vi "Sequencer.RF.vi"() -> ()   [LabVIEW 2014]
uses:
  <vilib>/Analysis/NI_AALPro.lvlib
panel:
  in  "Trigger":bool
  in  "Parameter":u16(ring) items=["Frequency (MHz)", "Amplitude (dBm)", "Phase (Pi)"]
  in  "Oscillators":u32(ring) items=["Agilent 1", "Agilent 2"]
  out "Counts":u32[](array[numeric])
  in  "Threshold":dbl=9.0
  out "CompiledSequence":string="#DopplerCooling\r\n0.9 10100000 00000000 00000000\r\n\r\n#Pump\r\n0.3 01000000 00000000 00000000\r\n\r\n#Pulsed\r\n0.2 00100000 00000000 00000000\r\n0.4 00000100 00000000 00000000\r\n0.2 00000000 10000000 00000000\r\n0.2 01000000 00000000 01000000\n"
  out "ChapterNames":string[](array[string])
  out "ChapterPositions":u32[](array[numeric])
  in  "Scan":enum32{"Time", "RF"}(tab)=enum."RF"
  out "Now (us)":dbl=1.0 format="%.2f"
  in  "Step (us)":dbl=1.0 format="%.2f"
  in  "End (us)":dbl=1.0 format="%.2f"
  in  "Start (us)":dbl=1.0 format="%.2f"
  in  "Time Scan":bool
  in  "Chapter":u16(ring) items=["Zero", "DopplerCooling", "OpticalPumping", "SinglePulseAWG", "Detection[0]", "Detection[1]", "Detection[2]", "Repump", "Zero"]
  in  "Once":bool=TRUE
  in  "Sequencer Port":refnum<visa-resource-name>="COM12"
  in  "Frequency (MHz)":dbl=1000.0 min=0.0 max=1000.0 step=1.0 format="%.3f"
  in  "Start":dbl=1.0 format="%.3f"
  in  "End":dbl=10.0 format="%.3f"
  in  "Step":dbl=0.1 format="%.3f"
  in  "Once":bool=TRUE
  in  "RF Scan":bool
  in  "RF":bool=TRUE
  in  "Amplitude (dBm)":dbl=-40.0 format="%.2f"
  in  "Phase (Pi)":dbl min=-1.0 max=1.0 step=0.1 format="%.2f"
  out "Durations Backup":dbl[](array[numeric])
  out "Durations":dbl[](array[numeric])
  in  "Period (ns)":dbl=5.0
  out "States":string[](array[string])
  in  "Sequencer":bool
  in  "Edit":enum32{"Sequence"}(tab)
  in  "Sequence":string
  in  "Save":bool
  in  "Chapter (us)":string
  in  "Sequence File":path=path "G:/Data/Sequence/Loading.seq"
  in  "Repeats":u32=100
  in  "Send":bool
  in  "Compile":bool
  out "Clock":string
  in  "Detect":enum32{"PMT", "TTL"}(tab)
  in  "4":bool=TRUE
  in  "3":bool=TRUE
  in  "2":bool=TRUE
  in  "1":bool=TRUE
  in  "Save":bool
  in  "Count or State":i16(ring) items=["Count", "State"]
  in  "Fit":bool
  out "Peak":u32
  out "?":cluster{dbl[], "Axis":dbl[]}(graph)
  out "?":cluster{"Axis":dbl[], "Histogram":i32[]}(graph)
  in  "Data Chapter":i16(ring) items=["All", "Repump"]
  out "Average Counts or States":dbl(graph)
  out "Average of Scans":dbl[](graph)
  out "data file":string
  out "History Data":dbl[](array[numeric])
  in  "Loop":bool
  in  "Clear":bool
  in  "Data":bool
  out "Digital Waveform Graph":digitaldata(graph)
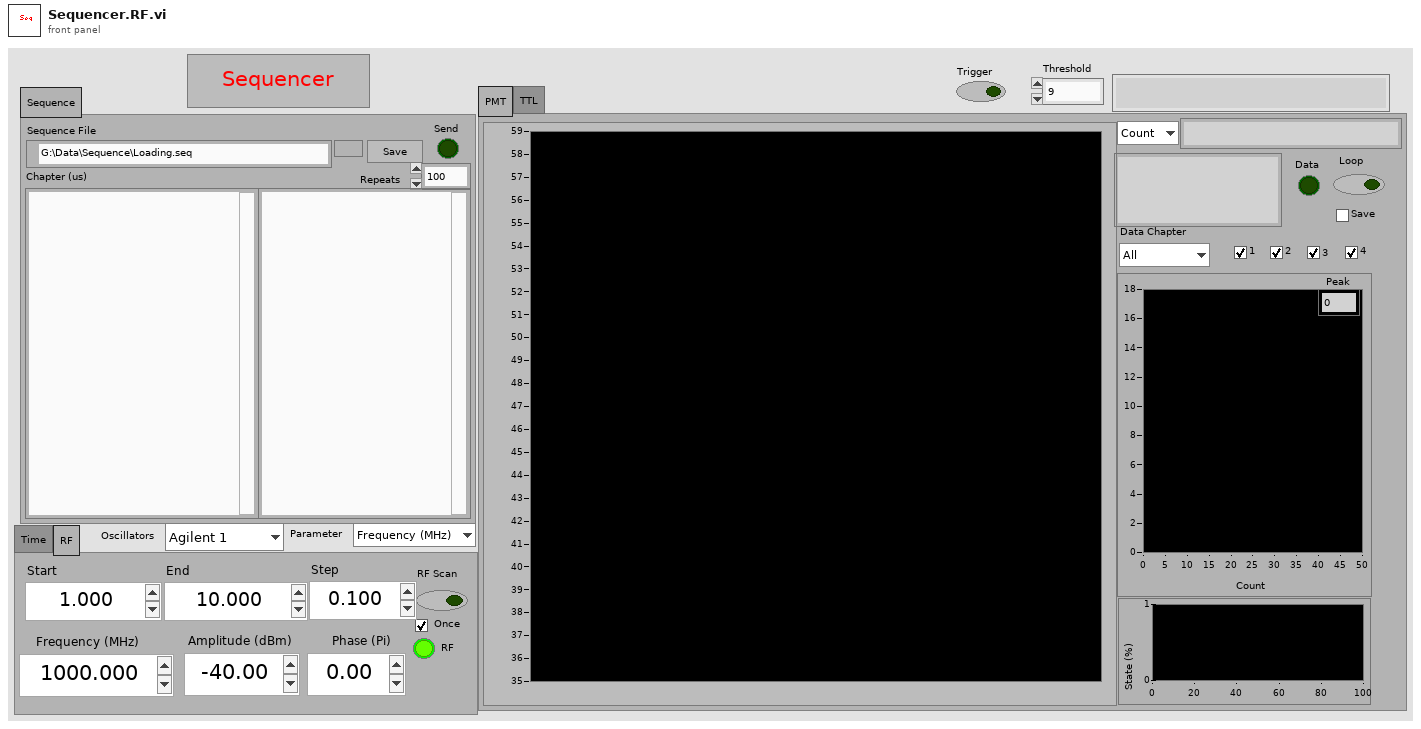
[diagram p1: front panel]
types:
  T1 = cluster{"lower":dbl, "upper":dbl, "inclusion":enum32{"lower", "upper", "both", "neither"}}[]
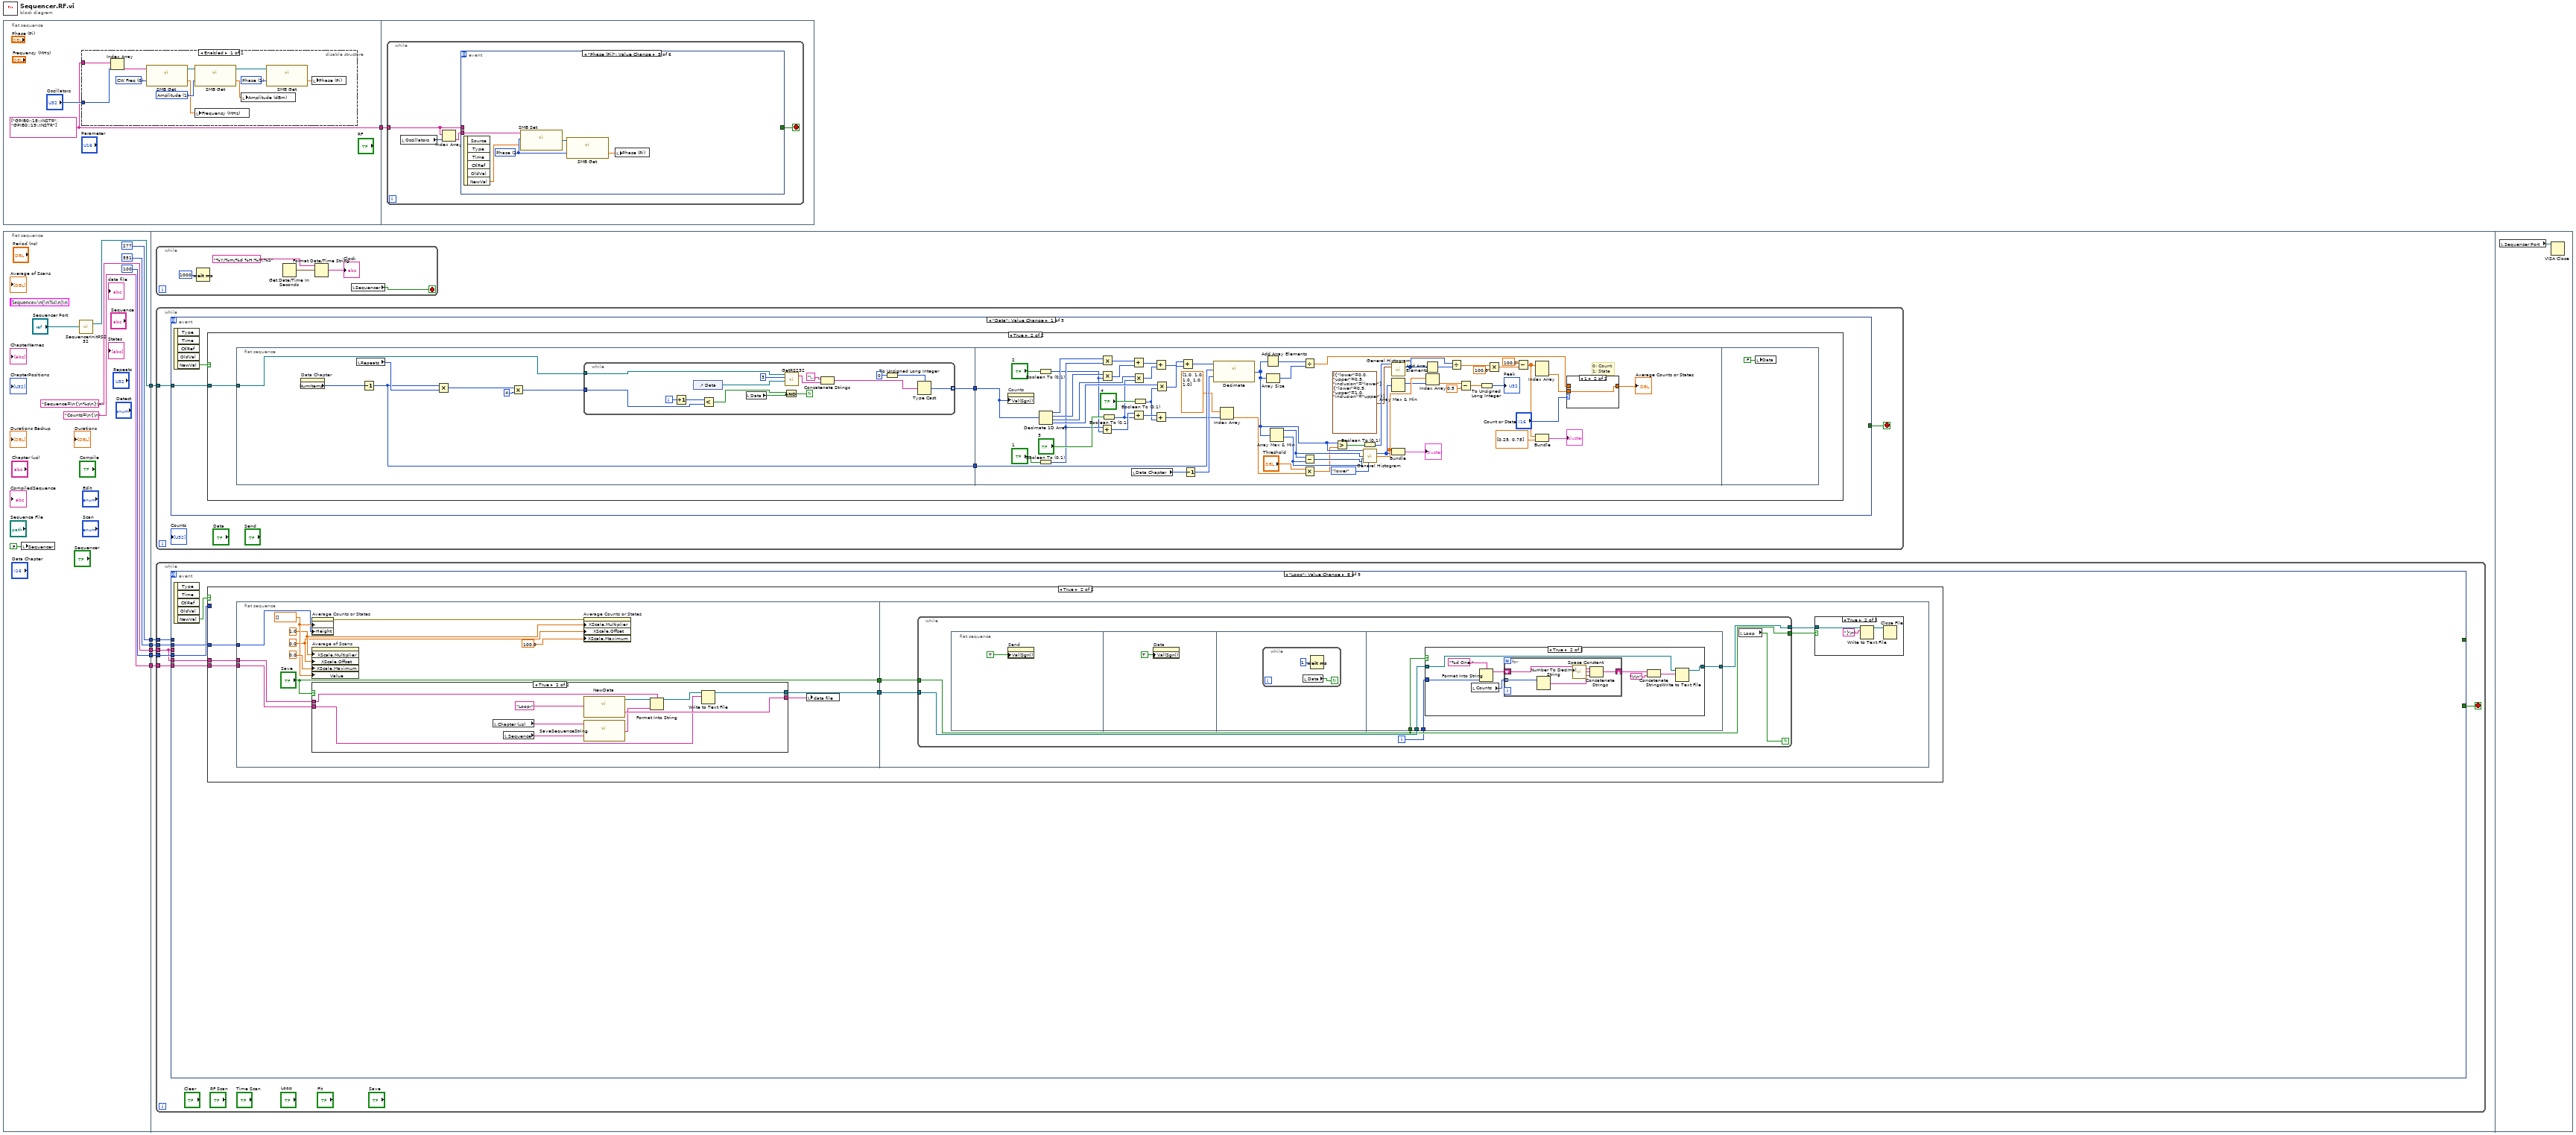
[diagram p0: block diagram]
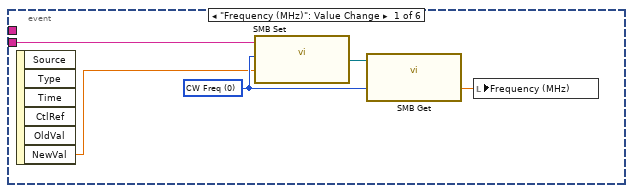
[diagram p3: hidden frame]
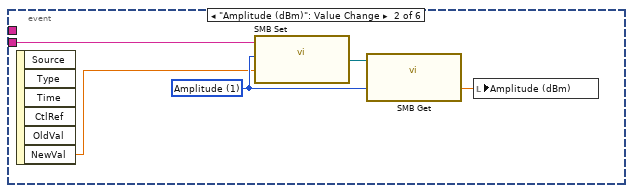
[diagram p4: hidden frame]
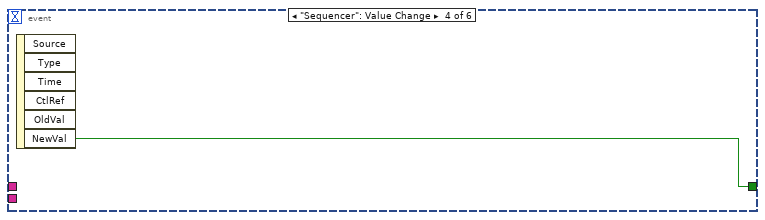
[diagram p5: hidden frame]
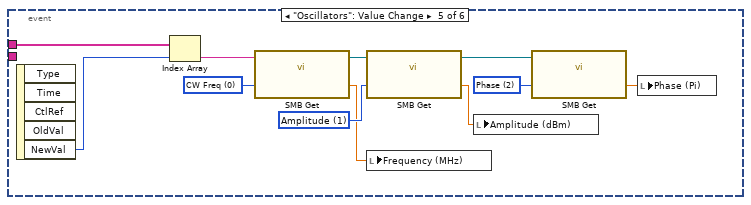
[diagram p6: hidden frame]
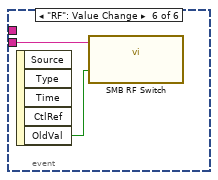
[diagram p7: hidden frame]
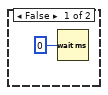
[diagram p8: hidden frame]
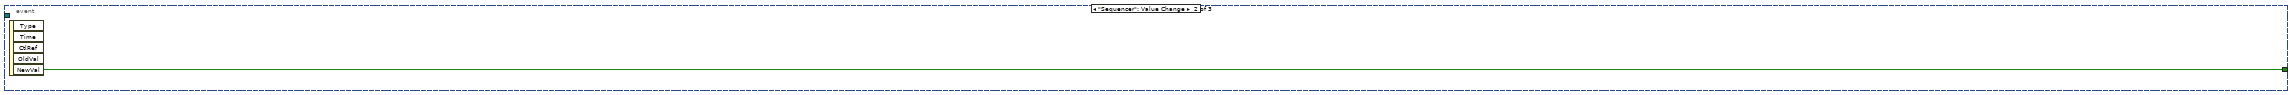
[diagram p10: hidden frame]
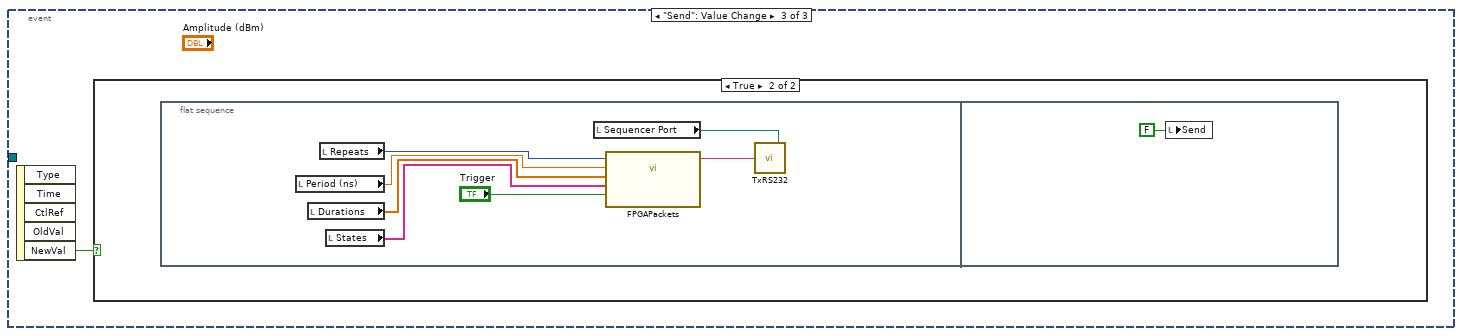
[diagram p11: hidden frame]
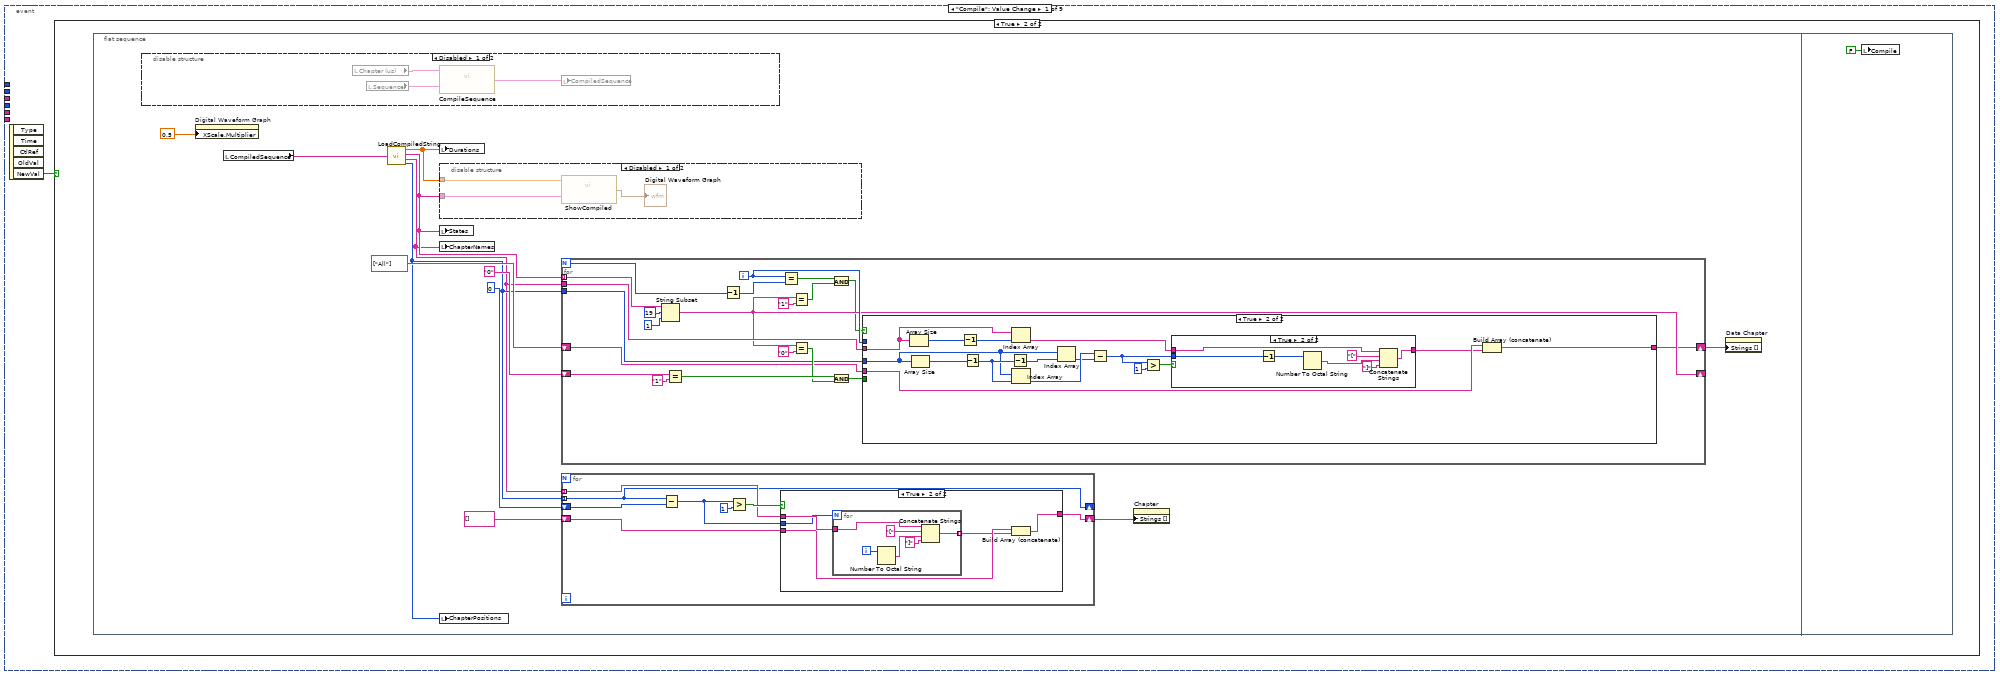
[diagram p13: hidden frame]
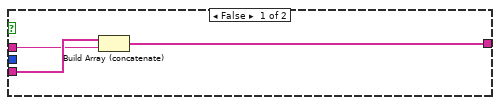
[diagram p17: hidden frame]
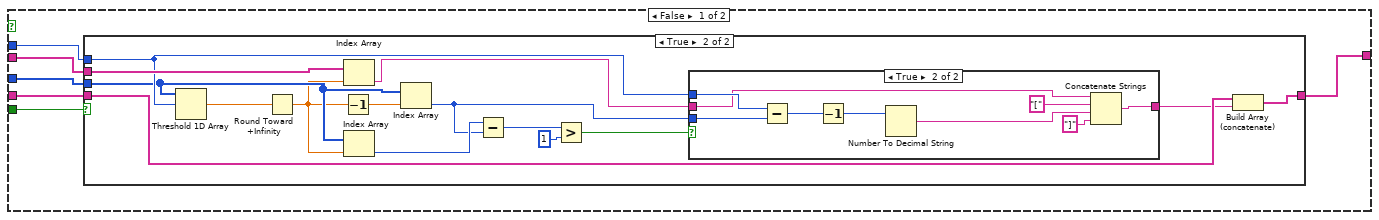
[diagram p18: hidden frame]
diagram:
  n1 = flat-sequence {
    tunnel: [w8] -> w1
    tunnel: w1 -> [w21]
    frame #0 {
      w8 = string[] ["GPIB0::18::INSTR", "GPIB0::19::INSTR"] ("array of strings")
      n2 = disable-structure shown="Enabled" {
        disable-tunnel: "Oscillators" -> [w20 _]
        disable-tunnel: w8 -> [w19 _]
        frame Enabled {
          w12 = u16 2 items=["CW Freq", "Amplitude", "Phase"] ("Ring")
          w15 = u16 1 items=["CW Freq", "Amplitude", "Phase"] ("Ring")
          w17 = u16 0 items=["CW Freq", "Amplitude", "Phase"] ("Ring")
          n3 = Index Array(array=w19, index=w20) -> (element=w18:string)
          n4 = call "SMB Get.vi"("Item"=w17, "VISA in"=w18) -> ("Value"=w10:dbl, "VISA out"=w16:refnum<visa-resource-name>)
          n5 = call "SMB Get.vi"("Item"=w15, "VISA in"=w16) -> ("Value"=w14:dbl, "VISA out"=w13:refnum<visa-resource-name>)
          n6 = local write "Frequency (MHz)"(w10) -> ()
          n7 = local write "Amplitude (dBm)"(w14) -> ()
          n8 = call "SMB Get.vi"("Item"=w12, "VISA in"=w13) -> ("Value"=w11:dbl)  [unwired: 1 out]
          n9 = local write "Phase (Pi)"(w11) -> ()
        }
        frame Disabled {
        }
      }
    }
    frame #1 {
      n10 = while {
        tunnel: w21 -> [w23]
        stop <- w25 stop-if-true
        n11 = local read "Oscillators"() -> (w24:u32)
        n12 = Index Array(array=w23, index=w24) -> (element=w22:string)
        n13 = event shown="[2] \"Phase (Pi)\": Value Change" {
          selector: _ -> [_ _ _ _ _ _]
          dyn-events: _ -> [_ _ _ _ _ _]
          timeout: _ -> [_ _ _ _ _ _]
          tunnel: [_ _ _ w41 _ _] -> w25
          tunnel: w23 -> [_ _ _ _ w52 _]
          tunnel: w22 -> [w30 w33 w37 _ _ w54]
          event "Frequency (MHz)": Value Change {
            w28 = u16 0 items=["CW Freq", "Amplitude", "Phase"] ("Item")
            n14 = event-data() -> ("NewVal"=w26:dbl)  [unwired: 6 out]
            n15 = call "SMB Set.vi"("Value"=w26, "Item"=w28, "VISA in"=w30) -> ("VISA out"=w29:refnum<visa-resource-name>)
            n16 = call "SMB Get.vi"("Item"=w28, "VISA in"=w29) -> ("Value"=w27:dbl)  [unwired: 1 out]
            n17 = local write "Frequency (MHz)"(w27) -> ()
          }
          event "Amplitude (dBm)": Value Change {
            w34 = u16 1 items=["CW Freq", "Amplitude", "Phase"] ("Item")
            n18 = event-data() -> ("NewVal"=w31:dbl)  [unwired: 6 out]
            n19 = call "SMB Set.vi"("Value"=w31, "Item"=w34, "VISA in"=w33) -> ("VISA out"=w35:refnum<visa-resource-name>)
            n20 = call "SMB Get.vi"("Item"=w34, "VISA in"=w35) -> ("Value"=w32:dbl)  [unwired: 1 out]
            n21 = local write "Amplitude (dBm)"(w32) -> ()
          }
          event "Phase (Pi)": Value Change {
            w39 = u16 2 items=["CW Freq", "Amplitude", "Phase"] ("Item")
            n22 = event-data() -> ("NewVal"=w36:dbl)  [unwired: 6 out]
            n23 = call "SMB Set.vi"("Value"=w36, "Item"=w39, "VISA in"=w37) -> ("VISA out"=w40:refnum<visa-resource-name>)
            n24 = call "SMB Get.vi"("Item"=w39, "VISA in"=w40) -> ("Value"=w38:dbl)  [unwired: 1 out]
            n25 = local write "Phase (Pi)"(w38) -> ()
          }
          event "Sequencer": Value Change {
            n26 = event-data() -> ("NewVal"=w41:bool)  [unwired: 6 out]
          }
          event "Oscillators": Value Change {
            w44 = u16 2 items=["CW Freq", "Amplitude", "Phase"] ("Ring")
            w48 = u16 1 items=["CW Freq", "Amplitude", "Phase"] ("Item")
            w49 = u16 0 items=["CW Freq", "Amplitude", "Phase"] ("Item")
            n27 = event-data() -> ("NewVal"=w51:u32)  [unwired: 5 out]
            n28 = Index Array(array=w52, index=w51) -> (element=w47:string)
            n29 = call "SMB Get.vi"("Item"=w49, "VISA in"=w47) -> ("Value"=w46:dbl, "VISA out"=w50:refnum<visa-resource-name>)
            n30 = call "SMB Get.vi"("Item"=w48, "VISA in"=w50) -> ("Value"=w45:dbl, "VISA out"=w43:refnum<visa-resource-name>)
            n31 = local write "Frequency (MHz)"(w46) -> ()
            n32 = local write "Amplitude (dBm)"(w45) -> ()
            n33 = call "SMB Get.vi"("Item"=w44, "VISA in"=w43) -> ("Value"=w42:dbl)  [unwired: 1 out]
            n34 = local write "Phase (Pi)"(w42) -> ()
          }
          event "RF": Value Change {
            n35 = event-data() -> ("OldVal"=w53:bool)  [unwired: 5 out]
            n36 = call "SMB RF Switch.vi"("state"=w53, "VISA in"=w54) -> ()  [unwired: 1 out]
          }
        }
      }
    }
  }
  n37 = flat-sequence {
    tunnel: [w55] -> w7
    tunnel: [u32 277 ("XControl:Container Bounds:Height")] -> w6
    tunnel: [u32 551 ("Plot Area:Size:Height")] -> w5
    tunnel: [100 ("y")] -> w4
    tunnel: ["Sequence=\n{\n%s\n}\n" ("format string")] -> w3
    tunnel: ["Counts=\n{\n" ("text")] -> w2
    tunnel: w7 -> [w68]
    tunnel: w6 -> [w67]
    tunnel: w5 -> [w66]
    tunnel: w4 -> [w65]
    tunnel: w3 -> [w64]
    tunnel: w2 -> [w63]
    frame #0 {
      n38 = local write "Sequencer"(FALSE ("Sequencer")) -> ()
      n39 = call "SequencerInitRS232.vi"("VISA resource name"="Sequencer Port") -> ("reference out"=w55:refnum<visa-resource-name>)  [unwired: 1 out]
    }
    frame #1 {
      n40 = while {
        stop <- w69 stop-if-true
        n41 = Wait (ms)(milliseconds to wait=u32 1000) -> ()  [unwired: 1 out]
        n42 = Get Date/Time In Seconds() -> (seconds since 1Jan1904=w73:timestamp)
        n43 = Format Date/Time String(time format string (%c)="%Y/%m/%d %H:%M:%S", seconds (now)=w73) -> (date/time string=→"Clock":string)  [unwired: 1 out]
        n44 = local read "Sequencer"() -> (w69:bool)
      }
      n45 = while {
        tunnel: w68 -> [w75]
        stop <- w74 stop-if-true
        n46 = event shown="[0] \"Data\": Value Change" {
          selector: _ -> [_ _ _]
          dyn-events: _ -> [_ _ _]
          timeout: _ -> [_ _ _]
          tunnel: w75 -> [w77 _ _]
          tunnel: [_ w169 _] -> w74
          event "Data": Value Change {
            n47 = event-data() -> ("NewVal"=w76:bool)  [unwired: 5 out]
            n48 = case shown="True" w76 {
              tunnel: w77 -> [_ w81]
              frame False {
                n49 = Wait (ms)(milliseconds to wait=u32 0) -> ()  [unwired: 1 out]
              }
              frame True {
                n50 = flat-sequence {
                  tunnel: w81 -> [w89]
                  tunnel: [w87] -> w80
                  tunnel: [w85] -> w79
                  tunnel: w80 -> [w134]
                  tunnel: w79 -> [w140]
                  frame #0 {
                    n51 = property on="Data Chapter" class="Ring (strict)"() -> ("NumItems"=w88:u32)  [unwired: 2 in, 2 out]
                    n52 = local read "Repeats"() -> (w86:u32)
                    n53 = Decrement(x=w88) -> (x-1=w85:u32)
                    n54 = Multiply(x=w85, y=w86) -> (x*y=w84:u32)
                    n55 = Multiply(x=w84, y=u32 4) -> (x*y=w83:u32)
                    n56 = while {
                      tunnel: w89 -> [w96]
                      tunnel: [w97] -> w87 mode=indexing
                      tunnel: w83 -> [w92]
                      i -> [w91]
                      stop <- w100 continue-if-true
                      n57 = Increment(x=w91) -> (x+1=w90:i32)
                      n58 = control-ref of="Data"() -> (w93:refnum<vi>)
                      n59 = Less?(x=w90, y=w92) -> (x < y?=w99:bool)
                      n60 = local read "Data"() -> (w101:bool)
                      n61 = And(x=w99, y=w101) -> (x .and. y?=w100:bool)
                      n62 = call "GetRS232.vi"("VISA resource name"=w96, "Bytes To Read"=3, "Control"=w93) -> ("Data"=w94:string)  [unwired: 2 in, 1 out]
                      n63 = Concatenate Strings("\u0000" ("string"), w94) -> (w98:string)
                      n64 = To Unsigned Long Integer(number=u32 0) -> (unsigned 32bit integer=w104:u32)
                      n65 = Type Cast(type=w104, x=w98) -> (*(type *) &x=w97:u32)
                    }
                  }
                  frame #1 {
                    # "0: Count\n1: State"
                    n66 = property on="Counts" class="Arr (strict)"("Val(Sgnl)"=w134) -> ()  [unwired: 2 in, 2 out]
                    n67 = Boolean To (0,1)(Boolean="2") -> (0, 1=w117:i16)
                    n68 = Boolean To (0,1)(Boolean="1") -> (0, 1=w118:i16)
                    n69 = Decimate 1D Array(w134) -> (w133:u32[], w130:u32[], w126:u32[], w123:u32[])
                    n70 = Add(x=w118, y=w117) -> (x+y=w116:i16)
                    n71 = Multiply(x=w133, y=w118) -> (x*y=w119:u32[])
                    n72 = Multiply(x=w130, y=w117) -> (x*y=w129:u32[])
                    n73 = Boolean To (0,1)(Boolean="3") -> (0, 1=w115:i16)
                    n74 = local read "Data Chapter"() -> (w138:i16)
                    n75 = Add(x=w119, y=w129) -> (x+y=w124:u32[])
                    n76 = Add(x=w116, y=w115) -> (x+y=w114:i16)
                    n77 = Multiply(x=w126, y=w115) -> (x*y=w125:u32[])
                    n78 = Boolean To (0,1)(Boolean="4") -> (0, 1=w113:i16)
                    n79 = Add(x=w124, y=w125) -> (x+y=w121:u32[])
                    n80 = Add(x=w114, y=w113) -> (x+y=w108:i16)
                    n81 = Multiply(x=w123, y=w113) -> (x*y=w122:u32[])
                    n82 = Add(x=w121, y=w122) -> (x+y=w120:u32[])
                    n83 = Decrement(x=w138) -> (x-1=w137:i16)
                    n84 = call "Decimate.vi"("i"=w137, "n"=w140, "Input Array"=w120) -> ("Decimated Array"=w162:u32[])
                    n85 = Index Array(array=dbl[] [1.0, 1.0, 1.0, 1.0, 1.0], index=w108) -> (element=w110:dbl)
                    n86 = Add Array Elements(numeric array=w162) -> (sum=w161:u32)
                    n87 = Array Size(array=w162) -> (size(s)=w160:i32)
                    n88 = Array Max & Min(array=w162) -> (max value=w141:u32, min value=w151:u32)  [unwired: 2 out]
                    n89 = Divide(x=w161, y=w160) -> (x/y=w163:dbl)
                    n90 = Subtract(x=w141, y=w151) -> (x-y=w150:u32)
                    n91 = Multiply(x="Threshold", y=w110) -> (x*y=w109:dbl)
                    n92 = Greater?(x=w162, y=w109) -> (0:w147:bool[])
                    n93 = Boolean To (0,1)(Boolean=w147) -> (0, 1=w146:i16[])
                    n94 = call <vilib>:"General Histogram.vi"("X"=w162, "max"=w141, "min"=w151, "# bins"=w150, "inclusion"=enum32{"lower", "upper"}."lower") -> ("Histogram"=w152:i32[], "Axis"=w154:dbl[])  [unwired: 1 in, 8 out]
                    n95 = call <vilib>:"General Histogram.vi"("X"=w146, "Bins"=T1 [{"lower"=0.0, "upper"=0.5, "inclusion"=enum."lower"}, {"lower"=0.5, "upper"=1.0, "inclusion"=enum."upper"}]) -> ("Histogram"=w144:i32[])  [unwired: 4 in, 9 out]
                    n96 = Array Max & Min(array=w152) -> (max index (indices)=w153:i32)  [unwired: 3 out]
                    n97 = Bundle("Axis"=w154, "Histogram"=w152) -> (→"?":cluster{"Axis":dbl[], "Histogram":i32[]})  [unwired: 1 out]
                    n98 = Add Array Elements(numeric array=w144) -> (sum=w145:i32)
                    n99 = Index Array(array=w154, index=w153) -> (element=w158:dbl)
                    n100 = Divide(x=w144, y=w145) -> (x/y=w142:dbl[])
                    n101 = Subtract(x=w158, y=0.5) -> (x-y=w157:dbl)
                    n102 = To Unsigned Long Integer(number=w157) -> (unsigned 32bit integer=→"Peak":u32)
                    n103 = Multiply(x=w142, y=100.0) -> (x*y=w106:dbl[])
                    n104 = Subtract(x=100.0 ("y"), y=w106) -> (x-y=w105:dbl[])
                    n105 = Index Array(array=w105) -> (element #2=w164:dbl)  [unwired: 2 in, 1 out]
                    n106 = Bundle(w105, "Axis"=dbl[] [0.25, 0.75]) -> (→"?":cluster{dbl[], "Axis":dbl[]})  [unwired: 1 out]
                    n107 = case shown="1" "Count or State" {
                      tunnel: w163 -> [w166 _]
                      tunnel: [w166 w167] -> w165
                      tunnel: w164 -> [_ w167]
                      frame 0, Default {
                      }
                      frame 1 {
                      }
                    }
                    "Average Counts or States" <- w165
                  }
                  frame #2 {
                    n108 = local write "Data"(FALSE ("Acquisition")) -> ()
                  }
                }
              }
            }
          }
          event "Sequencer": Value Change {
            n109 = event-data() -> ("NewVal"=w169:bool)  [unwired: 5 out]
          }
          event "Send": Value Change {
            n110 = event-data() -> ("NewVal"=w170:bool)  [unwired: 5 out]
            n111 = case shown="True" w170 {
              frame False {
              }
              frame True {
                n112 = flat-sequence {
                  frame #0 {
                    n113 = local read "Period (ns)"() -> (w175:dbl)
                    n114 = local read "Durations"() -> (w173:dbl[])
                    n115 = local read "Repeats"() -> (w174:u32)
                    n116 = local read "States"() -> (w176:string[])
                    n117 = local read "Sequencer Port"() -> (w177:refnum<visa-resource-name>)
                    n118 = call "FPGAPackets.vi"("Repeats"=w174, "Period (ns)"=w175, "Durations"=w173, "States"=w176, "Trigger"="Trigger") -> ("Packets"=w172:string)  [unwired: 1 out]
                    n119 = call "TxRS232.vi"("VISA resource name"=w177, "Data"=w172) -> ()
                  }
                  frame #1 {
                    n120 = local write "Send"(FALSE ("Send")) -> ()
                  }
                }
              }
            }
          }
        }
      }
      n121 = while {
        tunnel: w67 -> [w183]
        tunnel: w66 -> [w182]
        tunnel: w65 -> [w181]
        tunnel: w64 -> [w179]
        tunnel: w63 -> [w180]
        stop <- w184 stop-if-true
        n122 = event shown="[7] \"Loop\": Value Change" {
          selector: _ -> [_ _ _ _ _ _ _ _ _]
          dyn-events: _ -> [_ _ _ _ _ _ _ _ _]
          timeout: _ -> [_ _ _ _ _ _ _ _ _]
          tunnel: [_ _ _ _ _ _ _ _ w710] -> _
          tunnel: [_ _ _ _ _ _ _ _ w710] -> w184
          tunnel: w183 -> [_ w304 _ _ w490 _ _ _ _]
          tunnel: w182 -> [_ _ _ _ _ _ _ w645 _]
          tunnel: w181 -> [_ _ _ _ _ _ _ w644 _]
          tunnel: w179 -> [_ _ _ _ _ _ _ w643 _]
          tunnel: w180 -> [_ _ _ _ _ _ _ w642 _]
          tunnel: w179 -> [_ _ _ _ w489 _ _ _ _]
          event "Compile": Value Change {
            n123 = event-data() -> ("NewVal"=w185:bool)  [unwired: 5 out]
            n124 = case shown="True" w185 {
              frame False {
              }
              frame True {
                n125 = flat-sequence {
                  frame #0 {
                    n126 = disable-structure shown="Disabled" {
                      frame Disabled {
                        n127 = local read "Chapter (us)"() -> (w203:string)
                        n128 = local read "Sequence"() -> (w202:string)
                        n129 = call "CompileSequence.vi"("Sequence"=w202, "Chapter"=w203) -> ("Compiled Sequence"=w201:string)
                        n130 = local write "CompiledSequence"(w201) -> ()
                      }
                      frame Enabled {
                      }
                    }
                    n131 = property on="Digital Waveform Graph" class="DigitalGraph (strict)"("XScale.Multiplier"=0.5 ("X Scale.Offset and Multiplier:Multiplier")) -> ()  [unwired: 2 in, 2 out]
                    n132 = local read "CompiledSequence"() -> (w186:string)
                    n133 = call "LoadCompiledString.vi"("Compiled String"=w186) -> ("Durations"=w197:dbl[], "States"=w196:string[], "ChapterNames"=w187:string[], "ChapterPositions"=w188:u32[])
                    n134 = local write "Durations"(w197) -> ()
                    n135 = disable-structure shown="Disabled" {
                      disable-tunnel: w197 -> [w200 _]
                      disable-tunnel: w196 -> [w199 _]
                      frame Disabled {
                        n136 = call "ShowCompiled.vi"("States"=w199, "Durations"=w200) -> ("Digital Waveform Graph"=→"Digital Waveform Graph":digitaldata)
                      }
                      frame Enabled {
                      }
                    }
                    n137 = local write "States"(w196) -> ()
                    n138 = local write "ChapterNames"(w187) -> ()
                    n139 = local write "ChapterPositions"(w188) -> ()
                    n140 = for {
                      N -> [w236]
                      tunnel: w196 -> [w246] mode=indexing
                      shift-right: [w233] -> _
                      shift-left: "0" -> [w243]
                      tunnel: w187 -> [w239]
                      shift-right: [w228] -> w191
                      shift-left: string[] ["All"] -> [w227]
                      tunnel: w188 -> [w226]
                      i -> [w237]
                      n141 = String Subset(string=w246, offset (0)=19, length (rest)=1 ("length (rest)")) -> (substring=w233:string)
                      n142 = Equal?(x=w243, y="1") -> (x = y?=w241:bool)
                      n143 = Decrement(x=w236) -> (x-1=w235:i32)
                      n144 = Equal?(x=w237, y=w235) -> (x = y?=w232:bool)
                      n145 = Equal?(x=w233, y="1") -> (x = y?=w231:bool)
                      n146 = Equal?(x=w233, y="0") -> (x = y?=w238:bool)
                      n147 = And(x=w232, y=w231) -> (x .and. y?=w230:bool)
                      n148 = And(x=w241, y=w238) -> (x .and. y?=w229:bool)
                      n149 = case shown="True" w230 {
                        tunnel: w239 -> [w252 w292]
                        tunnel: w227 -> [w251 w294]
                        tunnel: w237 -> [w250 _]
                        tunnel: w229 -> [w249 _]
                        tunnel: [w248 w293] -> w228
                        tunnel: w226 -> [w247 w286]
                        frame False {
                          n150 = case shown="True" w249 {
                            tunnel: w250 -> [_ w264]
                            tunnel: w252 -> [_ w265]
                            tunnel: w251 -> [w253 w267]
                            tunnel: [w253 w268] -> w248
                            tunnel: w247 -> [_ w261]
                            frame False {
                            }
                            frame True {
                              n151 = Threshold 1D Array(2:w264, 3:w261) -> (0:w266:dbl)  [unwired: 1 out]
                              n152 = Round Toward +Infinity(x=w266) -> (ceil(x): smallest int >= x=w259:dbl)
                              n153 = Decrement(x=w259) -> (x-1=w260:dbl)
                              n154 = Index Array(array=w265, index=w259) -> (element=w262:string)
                              n155 = Index Array(array=w261, index=w259) -> (element=w258:u32)
                              n156 = Index Array(array=w261, index=w260) -> (element=w254:u32)
                              n157 = Subtract(x=w258, y=w254) -> (x-y=w257:u32)
                              n158 = Greater?(x=w257, y=u32 1) -> (0:w255:bool)
                              n159 = case shown="True" w255 {
                                tunnel: w264 -> [_ w278]
                                tunnel: [w269 w272] -> w263
                                tunnel: w262 -> [w269 w271]
                                tunnel: w254 -> [_ w270]
                                frame False {
                                }
                                frame True {
                                n160 = Subtract(x=w278, y=w270) -> (x-y=w277:u32)
                                n161 = Decrement(x=w277) -> (x-1=w276:u32)
                                n162 = Number To Decimal String(number=w276) -> (decimal integer string=w273:string)  [unwired: 1 out]
                                n163 = Concatenate Strings(w271, "[" ("element"), w273, "]" ("element")) -> (w272:string)
                                }
                              }
                              n164 = Build Array (concatenate)(w267, w263) -> (w268:string[])
                            }
                          }
                        }
                        frame True {
                          n165 = Array Size(array=w292) -> (size(s)=w291:i32)
                          n166 = Array Size(array=w286) -> (size(s)=w289:i32)
                          n167 = Decrement(x=w291) -> (x-1=w290:i32)
                          n168 = Decrement(x=w289) -> (x-1=w288:i32)
                          n169 = Decrement(x=w288) -> (x-1=w287:i32)
                          n170 = Index Array(array=w292, index=w290) -> (element=w281:string)
                          n171 = Index Array(array=w286, index=w288) -> (element=w285:u32)
                          n172 = Index Array(array=w286, index=w287) -> (element=w284:u32)
                          n173 = Subtract(x=w285, y=w284) -> (x-y=w279:u32)
                          n174 = Greater?(x=w279, y=u32 1) -> (0:w282:bool)
                          n175 = case shown="True" w282 {
                            tunnel: w281 -> [w295 w302]
                            tunnel: [w295 w296] -> w280
                            tunnel: w279 -> [_ w299]
                            frame False {
                            }
                            frame True {
                              n176 = Decrement(x=w299) -> (x-1=w298:u32)
                              n177 = Number To Octal String(2:w298) -> (0:w297:string)  [unwired: 1 out]
                              n178 = Concatenate Strings(w302, "[" ("string"), w297, "]" ("string")) -> (w296:string)
                            }
                          }
                          n179 = Build Array (concatenate)(w294, w280) -> (w293:string[])
                        }
                      }
                    }
                    n180 = for {
                      tunnel: w188 -> [w204] mode=indexing
                      tunnel: w187 -> [w205] mode=indexing
                      shift-right: [w204] -> _
                      shift-left: u32 0 ("initial scan location") -> [w211]
                      shift-right: [w206] -> w193
                      shift-left: string[] [] -> [w207]
                      n181 = Subtract(x=w204, y=w211) -> (x-y=w208:u32)
                      n182 = Greater?(x=w208, y=u32 1) -> (0:w210:bool)
                      n183 = case shown="True" w210 {
                        tunnel: w205 -> [w213 w219]
                        tunnel: w208 -> [_ w218]
                        tunnel: w207 -> [w214 w217]
                        tunnel: [w212 w215] -> w206
                        frame False {
                          n184 = Build Array (concatenate)(w214, w213) -> (w212:string[])
                        }
                        frame True {
                          n185 = for {
                            N: w218 -> [_]
                            tunnel: w219 -> [w224]
                            tunnel: [w223] -> w216 mode=indexing
                            i -> [w225]
                            n186 = Number To Octal String(2:w225) -> (0:w222:string)  [unwired: 1 out]
                            n187 = Concatenate Strings(w224, "[" ("string"), w222, "]" ("string")) -> (w223:string)
                          }
                          n188 = Build Array (concatenate)(w217, w216) -> (w215:string[])
                        }
                      }
                    }
                    n189 = property on="Chapter" class="Ring (strict)"("Strings []"=w193) -> ()  [unwired: 2 in, 2 out]
                    n190 = property on="Data Chapter" class="Ring (strict)"("Strings []"=w191) -> ()  [unwired: 2 in, 2 out]
                  }
                  frame #1 {
                    n191 = local write "Compile"(FALSE ("Compile")) -> ()
                  }
                }
              }
            }
          }
          event "RF Scan": Value Change {
            n192 = event-data() -> ("NewVal"=w305:bool)  [unwired: 6 out]
            n193 = case shown="True" w305 {
              tunnel: "Step" -> [_ w318]
              tunnel: "End" -> [_ w317]
              tunnel: "Start" -> [_ w313]
              tunnel: w304 -> [_ w316]
              frame False {
              }
              frame True {
                w319 = "\r\n"
                w347 = "\r\n"
                w350 = "\r\n"
                n194 = property on="Average of Scans" class="WFGraph (strict)"("XScale.Multiplier"=w318, "XScale.Offset"=w313, "XScale.Maximum"=w317) -> ()  [unwired: 2 in, 2 out]
                n195 = property on="Average Counts or States" class="WFChart (strict)"("Height"=w316, "History Data"=dbl[] []) -> (error out=w315:errorcluster)  [unwired: 2 in, 1 out]
                n196 = local read "Frequency (MHz)"() -> (w333:dbl)
                n197 = local read "Amplitude (dBm)"() -> (w329:dbl)
                n198 = local read "Chapter (us)"() -> (w367:string)
                n199 = local read "Parameter"() -> (w342:u16)
                n200 = local read "Phase (Pi)"() -> (w328:dbl)
                n201 = local read "Sequence"() -> (w366:string)
                n202 = local read "Start"() -> (w365:dbl)
                n203 = local read "Step"() -> (w356:dbl)
                n204 = local read "End"() -> (w309:dbl)
                n205 = call "SaveSequenceString.vi"("Sequence"=w366, "Chapter"=w367) -> ("Sequence String"=w362:string)
                n206 = property on="Parameter" class="Ring (strict)"() -> ("RingText.Text"=w320:string)  [unwired: 2 in, 2 out]
                n207 = Index Array(array=string[] [" MHz", " dBm", " Pi"] ("array of strings"), index=w342) -> (element=w341:string)
                n208 = Number To Fractional String(number=w333) -> (F-format string=w332:string)  [unwired: 3 out]
                n209 = Number To Fractional String(number=w329) -> (F-format string=w323:string)  [unwired: 3 out]
                n210 = Number To Fractional String(number=w328) -> (F-format string=w324:string)  [unwired: 3 out]
                n211 = Number To Fractional String(number=w309) -> (F-format string=w357:string)  [unwired: 3 out]
                n212 = Number To Fractional String(number=w356) -> (F-format string=w355:string)  [unwired: 3 out]
                n213 = Number To Fractional String(number=w365) -> (F-format string=w359:string)  [unwired: 3 out]
                n214 = property on="Average Counts or States" class="WFChart (strict)"(error in=w315, "XScale.Multiplier"=w318, "XScale.Offset"=w313, "XScale.Maximum"=w317) -> ()  [unwired: 1 in, 2 out]
                n215 = Subtract(x=w317, y=w313) -> (x-y=w369:dbl)
                n216 = Concatenate Strings("Frequency=" ("string"), w332, " MHz" ("string"), w319, "Amplitude=" ("string"), w323, " dBm" ("string"), w319, "Phase=" ("string"), w324, " Pi" ("string"), w319, "Parameter=" ("string"), w320, w319) -> (w331:string)
                n217 = Concatenate Strings("Start=" ("string"), w359, w341, w347, "End=" ("string"), w357, w341, w347, "Step=" ("string"), w355, w341, w347) -> (w345:string)
                n218 = Concatenate Strings("Sequence=" ("string"), w350, "{" ("string"), w350, w362, w350, "}" ("string"), w350) -> (w346:string)
                n219 = Concatenate Strings("Counts=" ("string"), w347, "{" ("string"), w347) -> (w344:string)
                n220 = Divide(x=w369, y=w318) -> (x/y=w368:dbl)
                n221 = call "NewData.vi"("Prefix"="RFScan-" ("string")) -> ("data file name"=w311:string, "data file refnum"=w310:refnum<file>)  [unwired: 2 in]
                n222 = Concatenate Strings(w346, w331, w345, w344) -> (w337:string)
                n223 = Increment(x=w368) -> (x+1=w340:dbl)
                n224 = local write "data file"(w311) -> ()
                n225 = Write to Text File(file (use dialog)=w310, text=w337) -> (refnum out=w336:refnum<file>)  [unwired: 1 in, 3 out]
                n226 = Initialize Array(0.0 ("element"), w340) -> (w335:dbl[])
                n227 = while {
                  tunnel: w342 -> [w390]
                  tunnel: w341 -> [w389]
                  tunnel: w318 -> [w388]
                  tunnel: w313 -> [w387]
                  tunnel: w317 -> [w386]
                  tunnel: w340 -> [w385]
                  shift-right: [w380] -> _
                  shift-left: w335 -> [w379]
                  tunnel: [w381] -> w339
                  tunnel: w336 -> [w377]
                  i -> [w378]
                  stop <- w371 continue-if-true
                  n228 = flat-sequence {
                    tunnel: w386 -> [w405]
                    tunnel: w387 -> [w406]
                    tunnel: w388 -> [w407]
                    tunnel: [w407] -> w393
                    tunnel: [w406] -> w392
                    tunnel: [w405] -> w391
                    tunnel: w377 -> [w418]
                    tunnel: w390 -> [w417]
                    tunnel: w389 -> [w416]
                    tunnel: w393 -> [w415]
                    tunnel: w392 -> [w414]
                    tunnel: w391 -> [_]
                    tunnel: w385 -> [w413]
                    tunnel: [w412] -> w375
                    tunnel: [w410] -> w374
                    tunnel: [w411] -> w373
                    tunnel: [w408] -> w372
                    tunnel: [w471] -> w376
                    tunnel: [w472] -> w381
                    tunnel: [w473] -> w383
                    tunnel: w375 -> [w470]
                    tunnel: w374 -> [w473]
                    tunnel: w373 -> [w472]
                    tunnel: w372 -> [w471]
                    tunnel: [w469] -> w371
                    frame #0 {
                      n229 = property on="Average Counts or States" class="WFChart (strict)"("History Data"=dbl[] []) -> ()  [unwired: 2 in, 2 out]
                    }
                    frame #1 {
                      n230 = To Unsigned Long Integer(number=w413) -> (unsigned 32bit integer=w410:u32)
                      n231 = Decrement(x=w410) -> (x-1=w409:u32)
                      n232 = while {
                        shift-right: [w435] -> _
                        shift-left: w414 -> [w434]
                        tunnel: w415 -> [w436]
                        shift-right: [w432] -> w411
                        shift-left: w418 -> [w433]
                        tunnel: w416 -> [w431]
                        tunnel: w417 -> [w430]
                        tunnel: [w427] -> w412
                        tunnel: w409 -> [w425]
                        tunnel: [w423] -> w408 mode=indexing
                        i -> [w426]
                        stop <- w428 continue-if-true
                        n233 = flat-sequence {
                          tunnel: w434 -> [w437]
                          tunnel: w430 -> [w438]
                          tunnel: [w437] -> w420
                          tunnel: w420 -> [w443]
                          tunnel: [w443] -> w419
                          tunnel: w419 -> [w445]
                          tunnel: [w445] -> w421
                          tunnel: w421 -> [w446]
                          tunnel: [w446] -> w422
                          tunnel: w422 -> [w448]
                          tunnel: [w448] -> w429
                          tunnel: w433 -> [w461]
                          tunnel: [w460] -> w432
                          tunnel: w431 -> [w455]
                          tunnel: w429 -> [w453]
                          tunnel: [w451] -> w423
                          frame #0 {
                            n234 = case shown="1" w438 {
                              tunnel: w437 -> [w439 w440 w441]
                              frame 0, Default {
                                n235 = property on="Frequency (MHz)" class="DigNum (strict)"("Val(Sgnl)"=w439) -> ()  [unwired: 2 in, 2 out]
                              }
                              frame 1 {
                                n236 = property on="Amplitude (dBm)" class="DigNum (strict)"("Val(Sgnl)"=w440) -> ()  [unwired: 2 in, 2 out]
                              }
                              frame 2 {
                                n237 = property on="Phase (Pi)" class="DigNum (strict)"("Val(Sgnl)"=w441) -> ()  [unwired: 2 in, 2 out]
                              }
                            }
                          }
                          frame #1 {
                            n238 = Wait (ms)(milliseconds to wait=u32 10) -> ()  [unwired: 1 out]
                          }
                          frame #2 {
                            n239 = property on="Send" class="Bool (strict)"("Val(Sgnl)"=TRUE ("Acquisition")) -> ()  [unwired: 2 in, 2 out]
                          }
                          frame #3 {
                            n240 = property on="Data" class="Bool (strict)"("Val(Sgnl)"=TRUE ("Acquisition")) -> ()  [unwired: 2 in, 2 out]
                          }
                          frame #4 {
                            n241 = while {
                              stop <- w450 continue-if-true
                              n242 = local read "Data"() -> (w450:bool)
                              n243 = Wait (ms)(milliseconds to wait=u32 1 ("等待时间（毫秒）")) -> ()  [unwired: 1 out]
                            }
                          }
                          frame #5 {
                            n244 = Number To Fractional String(number=w453) -> (F-format string=w462:string)  [unwired: 3 out]
                            n245 = local read "Counts"() -> (w452:u32[])
                            n246 = Concatenate Strings(w462, w455, "," ("string")) -> (w459:string)
                            n247 = for {
                              tunnel: w452 -> [w467] mode=indexing
                              shift-right: [w465] -> w458
                              shift-left: w459 -> [w464]
                              n248 = Number To Decimal String(number=w467) -> (decimal integer string=w466:string)  [unwired: 1 out]
                              n249 = call <vilib>:"Space Constant.vi"() -> ("String"=w463:string)
                              n250 = Concatenate Strings(w464, w463, w466) -> (w465:string)
                            }
                            n251 = local read "Average Counts or States"() -> (w451:dbl)
                            n252 = Concatenate Strings(w458, "\r\n") -> (w456:string)
                            n253 = Write to Text File(file (use dialog)=w461, text=w456) -> (refnum out=w460:refnum<file>)  [unwired: 1 in, 3 out]
                          }
                        }
                        n254 = Add(x=w434, y=w436) -> (x+y=w435:dbl)
                        n255 = local read "RF Scan"() -> (w427:bool)
                        n256 = Less?(x=w426, y=w425) -> (x < y?=w424:bool)
                        n257 = And(x=w424, y=w427) -> (x .and. y?=w428:bool)
                      }
                    }
                    frame #2 {
                      n258 = case shown="True" "Once" {
                        tunnel: w470 -> [w474 _]
                        tunnel: [w474 w475] -> w469
                        frame False {
                        }
                        frame True {
                          w475 = FALSE ("RF Scan")
                          n259 = local write "RF Scan"(w475) -> ()
                        }
                      }
                    }
                  }
                  n260 = Array Size(array=w376) -> (size(s)=w384:i32)
                  n261 = Equal?(x=w384, y=w383) -> (x = y?=w382:bool)
                  n262 = case shown="True" w382 {
                    tunnel: w378 -> [_ w399]
                    tunnel: [w394 w395] -> w380
                    tunnel: w376 -> [_ w398]
                    tunnel: w379 -> [w394 w397]
                    tunnel: w378 -> [_ w396]
                    frame False {
                    }
                    frame True {
                      n263 = Increment(x=w399) -> (x+1=w401:i32)
                      n264 = Divide(x=w397, y=w401) -> (x/y=w403:dbl[])
                      n265 = Divide(x=w398, y=w401) -> (x/y=w400:dbl[])
                      n266 = Multiply(x=w396, y=w403) -> (x*y=w402:dbl[])
                      n267 = Add(x=w402, y=w400) -> (x+y=w395:dbl[])
                      n268 = local write "Average of Scans"(w395) -> ()
                    }
                  }
                }
                n269 = Concatenate Strings("}" ("string"), "\r\n") -> (w338:string)
                n270 = Write to Text File(file (use dialog)=w339, text=w338) -> (refnum out=w353:refnum<file>)  [unwired: 1 in, 3 out]
                n271 = Close File(refnum=w353) -> ()  [unwired: 1 in, 2 out]
              }
            }
          }
          event "Clear": Value Change {
            n272 = event-data() -> ()  [unwired: 7 out]
            n273 = property on="Average Counts or States" class="WFChart (strict)"("History Data"=dbl[] []) -> ()  [unwired: 2 in, 2 out]
          }
          event "Save": Value Change {
            n274 = event-data() -> ("NewVal"=w477:bool)  [unwired: 5 out]
            n275 = case shown="True" w477 {
              frame False {
              }
              frame True {
                n276 = flat-sequence {
                  frame #0 {
                    n277 = local read "Sequence File"() -> (w482:path)
                    n278 = local read "Chapter (us)"() -> (w480:string)
                    n279 = local read "Sequence"() -> (w479:string)
                    n280 = call "SaveSequenceString.vi"("Sequence"=w479, "Chapter"=w480) -> ("Sequence String"=w481:string)
                    n281 = call "CompileSequence.vi"("Sequence"=w479, "Chapter"=w480) -> ("Compiled Sequence"=w478:string)
                    n282 = Not Equal?(x=w482, y=path "") -> (x != y?=w484:bool)
                    n283 = case shown="True" w484 {
                      tunnel: w482 -> [_ w486]
                      tunnel: w481 -> [_ w485]
                      frame False {
                      }
                      frame True {
                        n284 = Write to Text File(file (use dialog)=w486, text=w485) -> ()  [unwired: 1 in, 4 out]
                      }
                    }
                    n285 = local write "CompiledSequence"(w478) -> ()
                  }
                  frame #1 {
                    n286 = local write "Save"(FALSE ("Compile")) -> ()
                    n287 = property on="Compile" class="Bool (strict)"("Val(Sgnl)"=TRUE ("Value (Signaling)")) -> ()  [unwired: 2 in, 2 out]
                  }
                }
              }
            }
          }
          event "Time Scan": Value Change {
            n288 = event-data() -> ("NewVal"=w491:bool)  [unwired: 5 out]
            n289 = case shown="True" w491 {
              tunnel: w490 -> [_ w503]
              tunnel: w489 -> [_ w496]
              frame False {
                n290 = local read "Durations Backup"() -> (w492:dbl[])
                n291 = local write "Durations"(w492) -> ()
              }
              frame True {
                (unwired) "," ("delimiter (Tab)")
                w516 = " us" ("string")
                w513 = "\r\n"
                n292 = property on="Average Counts or States" class="WFChart (strict)"("Height"=w503, "History Data"=dbl[] []) -> (error out=w502:errorcluster)  [unwired: 2 in, 1 out]
                n293 = local read "Chapter (us)"() -> (w523:string)
                n294 = local read "Sequence"() -> (w524:string)
                n295 = property on="Average of Scans" class="WFGraph (strict)"("XScale.Multiplier"="Step (us)", "XScale.Offset"="Start (us)", "XScale.Maximum"="End (us)") -> ()  [unwired: 2 in, 2 out]
                n296 = Subtract(x="End (us)", y="Start (us)") -> (x-y=w531:dbl)
                n297 = Number To Decimal String(number="Chapter") -> (decimal integer string=w527:string)  [unwired: 1 out]
                n298 = Number To Fractional String(number="End (us)") -> (F-format string=w519:string)  [unwired: 3 out]
                n299 = Number To Fractional String(number="Start (us)") -> (F-format string=w521:string)  [unwired: 3 out]
                n300 = Number To Fractional String(number="Step (us)") -> (F-format string=w517:string)  [unwired: 3 out]
                n301 = call "NewData.vi"("Prefix"="TimeScan-" ("string")) -> ("data file name"=w500:string, "data file refnum"=w494:refnum<file>)  [unwired: 2 in]
                n302 = call "SaveSequenceString.vi"("Sequence"=w524, "Chapter"=w523) -> ("Sequence String"=w495:string)
                n303 = Divide(x=w531, y="Step (us)") -> (x/y=w530:dbl)
                n304 = property on="Average Counts or States" class="WFChart (strict)"(error in=w502, "XScale.Multiplier"="Step (us)", "XScale.Offset"="Start (us)", "XScale.Maximum"="End (us)") -> ()  [unwired: 1 in, 2 out]
                n305 = local write "data file"(w500) -> ()
                n306 = Concatenate Strings("Chapter=" ("string"), w527, w513, "Start=" ("string"), w521, w516, w513, "End=" ("string"), w519, w516, w513, "Step=" ("string"), w517, w516, w513, "Counts=" ("string"), w513, "{" ("string"), w513) -> (w525:string)
                n307 = Format Into String(format string=w496, initial string=w494, w495) -> (resulting string=w493:refnum<file>)  [unwired: 1 in, 1 out]
                n308 = Increment(x=w530) -> (x+1=w529:dbl)
                n309 = Write to Text File(file (use dialog)=w493, text=w525) -> (refnum out=w512:refnum<file>)  [unwired: 1 in, 3 out]
                n310 = local read "Durations"() -> (w506:dbl[])
                n311 = Initialize Array(0.0 ("element"), w529) -> (w505:dbl[])
                n312 = local write "Durations Backup"(w506) -> ()
                n313 = while {
                  tunnel: "Start (us)" -> [w557]
                  tunnel: "Step (us)" -> [w556]
                  tunnel: "End (us)" -> [w555]
                  shift-right: [w545] -> _
                  shift-left: w505 -> [w554]
                  tunnel: w529 -> [w541]
                  tunnel: "Chapter" -> [w544]
                  shift-right: [w543] -> w510
                  shift-left: w512 -> [w542]
                  tunnel: w506 -> [w540]
                  i -> [w547]
                  stop <- w533 continue-if-true
                  n314 = flat-sequence {
                    tunnel: w554 -> [w568]
                    tunnel: w555 -> [w569]
                    tunnel: w556 -> [w570]
                    tunnel: w557 -> [w571]
                    tunnel: [w571] -> w553
                    tunnel: [w570] -> w552
                    tunnel: [w569] -> w551
                    tunnel: [w568] -> w550
                    tunnel: w553 -> [w582]
                    tunnel: w552 -> [w581]
                    tunnel: w551 -> [_]
                    tunnel: w550 -> [w580]
                    tunnel: w544 -> [w578]
                    tunnel: w542 -> [w577]
                    tunnel: w540 -> [w575]
                    tunnel: w539 -> [w574]
                    tunnel: [w580] -> w537
                    tunnel: [w579] -> w536
                    tunnel: [w576] -> w535
                    tunnel: [w572] -> w534
                    tunnel: [w623] -> w538
                    tunnel: [w624] -> w543
                    tunnel: [w620] -> w533
                    tunnel: [w625] -> w546
                    tunnel: w537 -> [w625]
                    tunnel: w536 -> [w621]
                    tunnel: w535 -> [w624]
                    tunnel: w534 -> [w623]
                    frame #0 {
                      n315 = property on="Average Counts or States" class="WFChart (strict)"("History Data"=dbl[] []) -> ()  [unwired: 2 in, 2 out]
                    }
                    frame #1 {
                      n316 = Decrement(x=w574) -> (x-1=w573:u32)
                      n317 = while {
                        shift-right: [w595] -> _
                        shift-left: w582 -> [w583]
                        tunnel: w581 -> [w593]
                        tunnel: [w592] -> w579
                        tunnel: w578 -> [w589]
                        tunnel: w577 -> [w590]
                        tunnel: [w591] -> w576
                        tunnel: w575 -> [w588]
                        tunnel: w573 -> [w585]
                        tunnel: [w584] -> w572 mode=indexing
                        i -> [w587]
                        stop <- w594 continue-if-true
                        n318 = local read "Time Scan"() -> (w592:bool)
                        n319 = flat-sequence {
                          tunnel: w589 -> [w599]
                          tunnel: w583 -> [w598]
                          tunnel: w588 -> [w596]
                          tunnel: w583 -> [w612]
                          tunnel: w590 -> [w607]
                          tunnel: [w606] -> w591
                          tunnel: [w604] -> w584
                          frame #0 {
                            n320 = Replace Array Subset(array=w596, new element=w598, index=w599) -> (w597:dbl[])
                            n321 = local write "Durations"(w597) -> ()
                          }
                          frame #1 {
                            n322 = property on="Send" class="Bool (strict)"("Val(Sgnl)"=TRUE ("Acquisition")) -> ()  [unwired: 2 in, 2 out]
                          }
                          frame #2 {
                            n323 = property on="Data" class="Bool (strict)"("Val(Sgnl)"=TRUE ("Acquisition")) -> ()  [unwired: 2 in, 2 out]
                          }
                          frame #3 {
                            n324 = while {
                              stop <- w603 continue-if-true
                              n325 = local read "Data"() -> (w603:bool)
                              n326 = Wait (ms)(milliseconds to wait=u32 1 ("等待时间（毫秒）")) -> ()  [unwired: 1 out]
                            }
                          }
                          frame #4 {
                            n327 = Number To Fractional String(number=w612) -> (F-format string=w614:string)  [unwired: 3 out]
                            n328 = local read "Counts"() -> (w605:u32[])
                            n329 = Concatenate Strings(w614, " us," ("string")) -> (w611:string)
                            n330 = for {
                              tunnel: w605 -> [w619] mode=indexing
                              shift-right: [w617] -> w608
                              shift-left: w611 -> [w616]
                              n331 = Number To Decimal String(number=w619) -> (decimal integer string=w618:string)  [unwired: 1 out]
                              n332 = call <vilib>:"Space Constant.vi"() -> ("String"=w615:string)
                              n333 = Concatenate Strings(w616, w615, w618) -> (w617:string)
                            }
                            n334 = Concatenate Strings(w608, "\r\n") -> (w609:string)
                            n335 = local read "Average Counts or States"() -> (w604:dbl)
                            n336 = Write to Text File(file (use dialog)=w607, text=w609) -> (refnum out=w606:refnum<file>)  [unwired: 1 in, 3 out]
                          }
                        }
                        n337 = Add(x=w583, y=w593) -> (x+y=w595:dbl)
                        n338 = Less?(x=w587, y=w585) -> (x < y?=w586:bool)
                        n339 = And(x=w592, y=w586) -> (x .and. y?=w594:bool)
                        "Now (us)" <- w583
                      }
                    }
                    frame #2 {
                      n340 = case shown="True" "Once" {
                        tunnel: w621 -> [w626 _]
                        tunnel: [w626 w628] -> w620
                        frame False {
                        }
                        frame True {
                          w628 = FALSE ("Time Scan")
                          n341 = local read "Durations Backup"() -> (w627:dbl[])
                          n342 = local write "Durations"(w627) -> ()
                          n343 = local write "Time Scan"(w628) -> ()
                        }
                      }
                    }
                  }
                  n344 = To Unsigned Long Integer(number=w541) -> (unsigned 32bit integer=w539:u32)
                  n345 = Array Size(array=w538) -> (size(s)=w548:i32)
                  n346 = Equal?(x=w548, y=w539) -> (x = y?=w549:bool)
                  n347 = case shown="True" w549 {
                    tunnel: w547 -> [_ w562]
                    tunnel: w538 -> [_ w561]
                    tunnel: w546 -> [w558 w560]
                    tunnel: [w558 w559] -> w545
                    frame False {
                    }
                    frame True {
                      n348 = Increment(x=w562) -> (x+1=w565:i32)
                      n349 = Divide(x=w561, y=w565) -> (x/y=w566:dbl[])
                      n350 = Divide(x=w562, y=w565) -> (x/y=w563:dbl)
                      n351 = Multiply(x=w560, y=w563) -> (x*y=w564:dbl[])
                      n352 = Add(x=w564, y=w566) -> (x+y=w559:dbl[])
                      n353 = local write "Average of Scans"(w559) -> ()
                    }
                  }
                }
                n354 = Concatenate Strings("}" ("string"), "\r\n") -> (w507:string)
                n355 = Write to Text File(file (use dialog)=w510, text=w507) -> (refnum out=w511:refnum<file>)  [unwired: 1 in, 3 out]
                n356 = Close File(refnum=w511) -> ()  [unwired: 1 in, 2 out]
              }
            }
          }
          event "Fit": Value Change {
            n357 = event-data() -> ("NewVal"=w629:bool)  [unwired: 5 out]
            n358 = case shown="True" w629 {
              frame False {
              }
              frame True {
                n359 = local write "Fit"(FALSE ("Fit")) -> ()
                n360 = property on="Average Counts or States" class="WFChart (strict)"() -> ("History Data"=→"History Data":dbl[])  [unwired: 2 in, 2 out]
              }
            }
          }
          event "Sequence File": Value Change {
            n361 = event-data() -> ("NewVal"=w633:path)  [unwired: 5 out]
            n362 = call <vilib>:"Check if File or Folder Exists.vi"("path"=w633) -> ("file or folder exists?"=w634:bool, "dup path"=w632:path)  [unwired: 1 in, 8 out]
            n363 = case shown="True" w634 {
              tunnel: w632 -> [_ w635]
              frame False {
              }
              frame True {
                n364 = flat-sequence {
                  tunnel: w635 -> [w639]
                  frame #0 {
                    n365 = Read from Text File(file (use dialog)=w639) -> (text=w640:string)  [unwired: 1 in, 5 out]
                    n366 = call "LoadSequenceString.vi"("Sequence String"=w640) -> ("Chapter"=w638:string, "Sequence"=w637:string)
                    n367 = local write "Chapter (us)"(w638) -> ()
                    n368 = call "CompileSequence.vi"("Sequence"=w637, "Chapter"=w638) -> ("Compiled Sequence"=w636:string)
                    n369 = local write "Sequence"(w637) -> ()
                    n370 = local write "CompiledSequence"(w636) -> ()
                  }
                  frame #1 {
                    n371 = property on="Compile" class="Bool (strict)"("Val(Sgnl)"=TRUE ("Value (Signaling)")) -> ()  [unwired: 2 in, 2 out]
                  }
                }
              }
            }
          }
          event "Loop": Value Change {
            n372 = event-data() -> ("NewVal"=w646:bool)  [unwired: 5 out]
            n373 = case shown="True" w646 {
              tunnel: w645 -> [_ w651]
              tunnel: w644 -> [_ _]
              tunnel: w643 -> [_ w650]
              tunnel: w642 -> [_ w649]
              frame False {
              }
              frame True {
                n374 = flat-sequence {
                  tunnel: w651 -> [w661]
                  tunnel: w650 -> [w656]
                  tunnel: w649 -> [w655]
                  tunnel: [w654] -> w648
                  tunnel: ["Save"] -> w647
                  tunnel: w648 -> [w678]
                  tunnel: w647 -> [w676]
                  frame #0 {
                    w662 = dbl[] [] ("History Data")
                    w659 = 0.0 ("X Scale.Offset and Multiplier:Offset")
                    w660 = 1.0 ("X Scale.Offset and Multiplier:Multiplier")
                    n375 = property on="Average Counts or States" class="WFChart (strict)"("History Data"=w662, "Height"=w661) -> (error out=w657:errorcluster)  [unwired: 2 in, 1 out]
                    n376 = property on="Average of Scans" class="WFGraph (strict)"("XScale.Multiplier"=w660, "XScale.Offset"=w659, "XScale.Maximum"=0.0 ("X Scale.Range:Maximum"), "Value"=w662) -> ()  [unwired: 2 in, 2 out]
                    n377 = case shown="True" "Save" {
                      tunnel: ["" w673] -> w653
                      tunnel: w656 -> [_ w670]
                      tunnel: w655 -> [_ w667]
                      tunnel: [_ w666] -> w654
                      frame False {
                      }
                      frame True {
                        n378 = local read "Chapter (us)"() -> (w672:string)
                        n379 = local read "Sequence"() -> (w668:string)
                        n380 = call "NewData.vi"("Prefix"="Loop-") -> ("data file name"=w673:string, "data file refnum"=w671:refnum<file>)  [unwired: 2 in]
                        n381 = call "SaveSequenceString.vi"("Sequence"=w668, "Chapter"=w672) -> ("Sequence String"=w669:string)
                        n382 = Format Into String(format string=w670, initial string=w671, w669) -> (resulting string=w665:refnum<file>)  [unwired: 1 in, 1 out]
                        n383 = Write to Text File(file (use dialog)=w665, text=w667) -> (refnum out=w666:refnum<file>)  [unwired: 1 in, 3 out]
                      }
                    }
                    n384 = property on="Average Counts or States" class="WFChart (strict)"(error in=w657, "XScale.Multiplier"=w660, "XScale.Offset"=w659, "XScale.Maximum"=100.0 ("X Scale.Range:Maximum")) -> ()  [unwired: 1 in, 2 out]
                    n385 = local write "data file"(w653) -> ()
                  }
                  frame #1 {
                    n386 = while {
                      tunnel: [w685] -> w677
                      tunnel: w678 -> [w684]
                      tunnel: w676 -> [w683]
                      tunnel: [w683] -> w675
                      i -> [w682]
                      stop <- w686 continue-if-true
                      n387 = flat-sequence {
                        tunnel: [w694] -> w685
                        tunnel: w684 -> [w693]
                        tunnel: w683 -> [w692]
                        tunnel: w682 -> [w691]
                        frame #0 {
                          n388 = property on="Send" class="Bool (strict)"("Val(Sgnl)"=TRUE ("Value (Signaling)")) -> ()  [unwired: 2 in, 2 out]
                        }
                        frame #1 {
                          n389 = property on="Data" class="Bool (strict)"("Val(Sgnl)"=TRUE ("Value (Signaling)")) -> ()  [unwired: 2 in, 2 out]
                        }
                        frame #2 {
                          n390 = while {
                            stop <- w690 continue-if-true
                            n391 = local read "Data"() -> (w690:bool)
                            n392 = Wait (ms)(milliseconds to wait=u32 1 ("等待时间（毫秒）")) -> ()  [unwired: 1 out]
                          }
                        }
                        frame #3 {
                          n393 = case shown="True" w692 {
                            tunnel: [w695 w700] -> w694
                            tunnel: w693 -> [w695 w699]
                            tunnel: w691 -> [_ w696]
                            frame False {
                            }
                            frame True {
                              n394 = local read "Counts"() -> (w704:u32[])
                              n395 = Format Into String(format string="%d One,", w696) -> (resulting string=w697:string)  [unwired: 2 in, 1 out]
                              n396 = for {
                                tunnel: w704 -> [w709] mode=indexing
                                shift-right: [w707] -> w703
                                shift-left: w697 -> [w706]
                                n397 = Number To Decimal String(number=w709) -> (decimal integer string=w708:string)  [unwired: 1 out]
                                n398 = call <vilib>:"Space Constant.vi"() -> ("String"=w705:string)
                                n399 = Concatenate Strings(w706, w705, w708) -> (w707:string)
                              }
                              n400 = Concatenate Strings(w703, "\r\n") -> (w701:string)
                              n401 = Write to Text File(file (use dialog)=w699, text=w701) -> (refnum out=w700:refnum<file>)  [unwired: 1 in, 3 out]
                            }
                          }
                        }
                      }
                      n402 = local read "Loop"() -> (w686:bool)
                    }
                    n403 = case shown="True" w675 {
                      tunnel: w677 -> [_ w680]
                      frame False {
                      }
                      frame True {
                        n404 = Write to Text File(file (use dialog)=w680, text="}\n") -> (refnum out=w681:refnum<file>)  [unwired: 1 in, 3 out]
                        n405 = Close File(refnum=w681) -> ()  [unwired: 1 in, 2 out]
                      }
                    }
                  }
                }
              }
            }
          }
          event "Sequencer": Value Change {
            n406 = event-data() -> ("NewVal"=w710:bool)  [unwired: 5 out]
          }
        }
      }
    }
    frame #2 {
      n407 = local read "Sequencer Port"() -> (w711:refnum<visa-resource-name>)
      n408 = VISA Close(VISA resource name=w711) -> ()  [unwired: 1 in, 1 out]
    }
  }
